vi "VISAuntitledStuff.vi"() -> ()   [LabVIEW 2009]
uses:
  <instrlib>/Agilent 546XX Series/Agilent 546XX Series.lvlib
panel:
  out "error out 2":errorcluster caption="error out" {"code" format="%.0x"}
  out "error out":errorcluster {"code" format="%.0x"}
  out "output waveform":waveform(dbl)
  in  "Serial Configuration":cluster{"Baud Rate":u32, "Flow Control":u16}={"Baud Rate"=0, "Flow Control"=4} {"Flow Control" items=["None", "XON/XOFF", "RTS/CTS", "XON/XOFF & RTS/CTS", "DTR/DSR", "XON/XOFF & DTR/DSR"]; "Baud Rate" items=["9600", "19200", "38400", "57600"]}
  in  "VISA Resource Name":refnum<visa-resource-name>="GPIB0::7::INSTR"
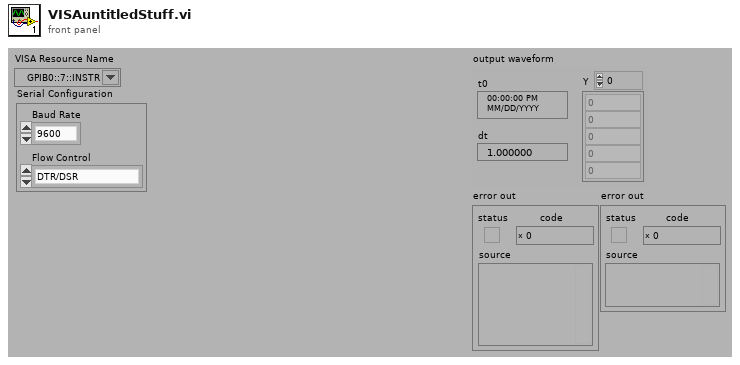
[diagram p1: front panel]
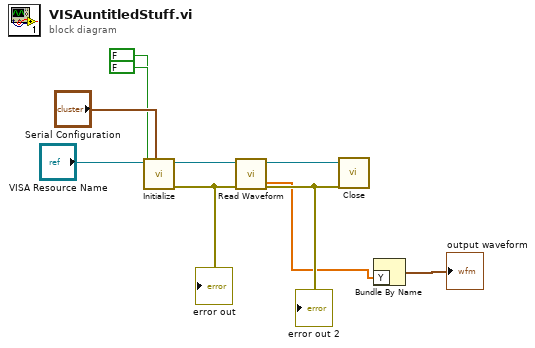
[diagram p0: block diagram]
diagram:
  n1 = call <instrlib>:"Initialize.vi"("Serial Configuration"="Serial Configuration", "ID Query (T: Query)"=FALSE, "Reset Device (T: Reset)"=FALSE, "VISA Resource Name"="VISA Resource Name") -> ("error out"=w7:errorcluster, "VISA Resource Name Out"=w8:refnum<visa-resource-name>)  [unwired: 6 in]
  "error out" <- w7
  n2 = call <instrlib>:"Read Waveform.vi"("error in (no error)"=w7, "VISA Resource Name"=w8) -> ("error out"=w6:errorcluster, "VISA Resource Name Out"=w5:refnum<visa-resource-name>, "waveform array"=w4:dbl[])  [unwired: 4 in, 3 out]
  "error out 2" <- w6
  n3 = call <instrlib>:"Close.vi"("error in (no error)"=w6, "VISA Resource Name"=w5) -> ()  [unwired: 9 in, 1 out]
  n4 = Bundle By Name("Y"=w4) -> (→"output waveform":waveform(dbl))  [unwired: 1 in]
